vi "Real time state machine - Saccade suppression LED by time.vi"() -> ()   [LabVIEW 2013]
uses:
  <vilib>/Platform/TimedLoop/XDataNode/timing_clust.ctl
  <vilib>/Platform/TimedLoop/XDataNode/nitl_modes.ctl
  <vilib>/Platform/TimedLoop/XDataNode/wakeup.ctl
  <vilib>/DAQmx/write.llb/DAQmx Write (Digital 1D Bool NChan 1Samp 1Line).vi
  <vilib>/DAQmx/read.llb/DAQmx Read (Analog 1D DBL NChan 1Samp).vi
  <vilib>/DAQmx/write.llb/DAQmx Write (Analog DBL 1Chan 1Samp).vi
  <vilib>/platform/TimedLoop/XDataNode/XDataNode.xnode
  <vilib>/Platform/TimedLoop/XDataNode/XDNodeRunTimeDep.lvlib
panel:
  in  "Local port":u16=9091
  in  "Local IP_This computer":string="192.168.137.2"
  out "ABORT":bool
  out "Initial data received":bool
  out "Busy":bool
  out "Trial Done":bool
  in  "Remote port":u16=9090
  in  "Remote IP_Main":string="192.168.137.10"
  out "Trial #":i32=1
  out "Start one trial":bool
  out "RT FIFO (Log)":u32(slide) scale=0.0..50.0
  out "error out":errorcluster
  out "Actual cycle period (uS)":i64=94
  out "# of rewards":i32
  in  "Automatic reward":bool=TRUE
  out "Digital Waveform Graph":digitalwaveform(graph)={"t0"=timestamp(3524542772.3366966 s since 1904-01-01), "dt"=0.0004, "Y"={"transitions"=[], "data"=array25000x3[75000 elements]}, "error"={"status"=FALSE, "code"=37421928, "source"=""}}
  out "shaft encoder":waveform(sgl)(graph)={"t0"=timestamp(3524542772.3366966 s since 1904-01-01), "dt"=0.02, "Y"=array[500 elements]}
  out "Min":dbl
  out "Sec":dbl=47.16078567504883
  out "Trial # (State machine)":u32=1
  out "Current state":T1(ring)=enum."VS"
  out "RT FIFO (DISP)":u32(slide) scale=0.0..50.0
  in  "State machine cycle (uS)":i64=200
  in  "Save file to":string="C:\\ni-rt\\LabVIEW Data\\"
  in  "Display length (S)":sgl=10.0
  in  "RT FIFO size":u32=50
  in  "VS filter period (uS)":i32=500
  out "LED?":bool
  out "Pulse amp 0":sgl
  out "Pulse amp 1":sgl
  out "Pulse delay":sgl
  out "Pulse width":sgl
  out "Pulse period (ms)":sgl
  out "Pulse #":sgl
  out "Reward period (uS)":u32
  out "Reward start delay (uS)":u32
  out "Water duration (uS)":u32=30000
  out "Water refractory period (uS)":u32=500000
  out "Shock duration (uS)":u32=10000
  out "Shock refractory period (uS)":u32=1000000
  out "Trial timeout (uS)":u32=3000000
  out "Lick threshold (V)":fxp<+,32,16>=1.600006103515625
  out "Track eye":bool=TRUE
  out "Allow shock":bool
  out "Allow timeout":bool
  out "Manually give water":bool
  out "Manually give shock":bool
  out "VS threshold (V)":fxp<+,32,16>=0.5
  out "VS type":string="continuous_flash"
  out "File name":string="Test"
  out "Behavior type":string="fullfield"
  out "Save data":bool
  out "Lick reward":bool
  in  "Stop state":bool
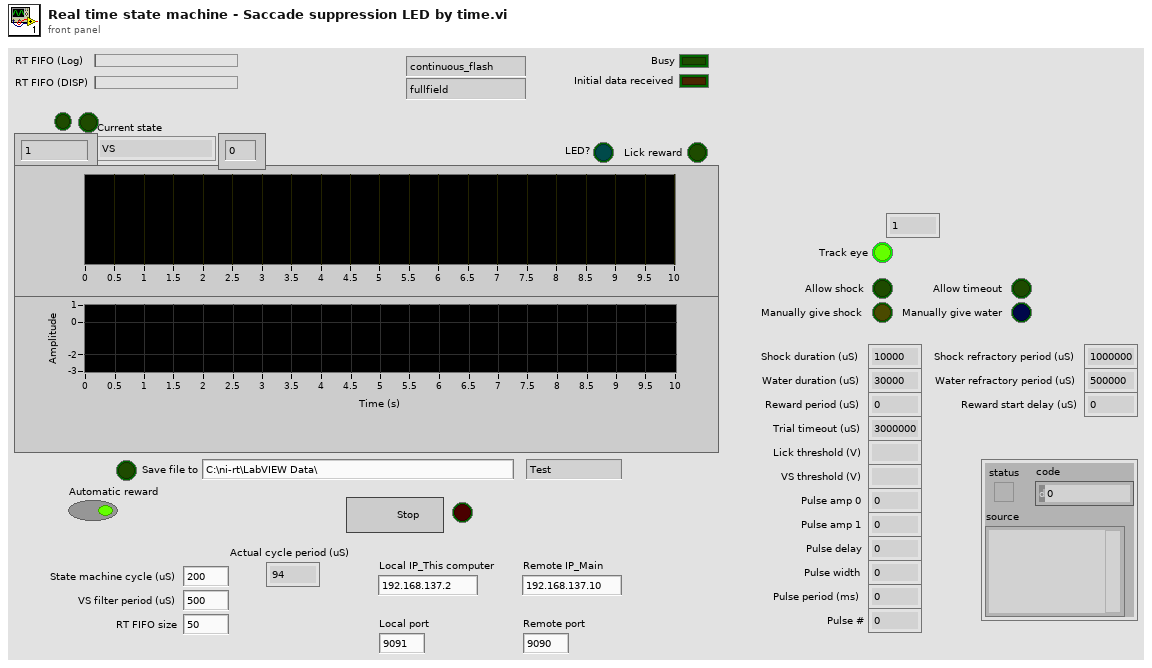
[diagram p1: front panel]
types:
  T1 = enum16{"Idle", "Before VS", "VS", "VS2", "After VS", "Wait for lever press", "Cycle End", "Reward", "Reward Refractory", "Punish", "Punish Refractory", "Exit", "Timeout", "Lick reward"}
  T2 = enum16{"open", "replace", "create", "open or create", "replace or create", "replace or create with confirmation"}
  T3 = typedef "XDNodeRunTimeDep.lvlib/timing_clust.ctl" = cluster{"Expected End [f-1]":u64, "Actual End [f-1]":u64, "Finished Late? [f-1]":bool, "Expected End [i-1]":u64, "Actual End [i-1]":u64, "Finished Late? [i-1]":bool, "Expected Start [i]":u64, "Actual Start [i]":u64, "Expected Start [f]":u64, "Actual Start [f]":u64, "Source Name":string, "Structure Name":string, "Period":i64, "Deadline":i64, "Offset":i64, "Start":i64, "Priority":i32, "Timeout":i32, "Mode":T4, "Wakeup Reason":T5, "Error":errorcluster, "Source Type":string, "Secondary Source Type":string, "Global End Time":u64, "Global Start Time":u64, "Frame Duration":u64, "Iteration Duration":u64, "Assigned CPU":i32, "I/O Scan Engine Mode":u32}
  T4 = typedef "XDNodeRunTimeDep.lvlib/nitl_modes.ctl" = enum32{"No Change", "Process missed periods, maintain original phase", "Discard missed periods, maintain original phase", "Process missed periods, ignore original phase", "Discard missed periods, ignore original phase"}
  T5 = typedef "XDNodeRunTimeDep.lvlib/wakeup.ctl" = enum32{"Normal", "Aborted", "Asynchronous wakeup", "Timing source error", "Timed loop error", "Timeout"}
  T6 = enum16{"big-endian, network order", "native, host order", "little-endian"}
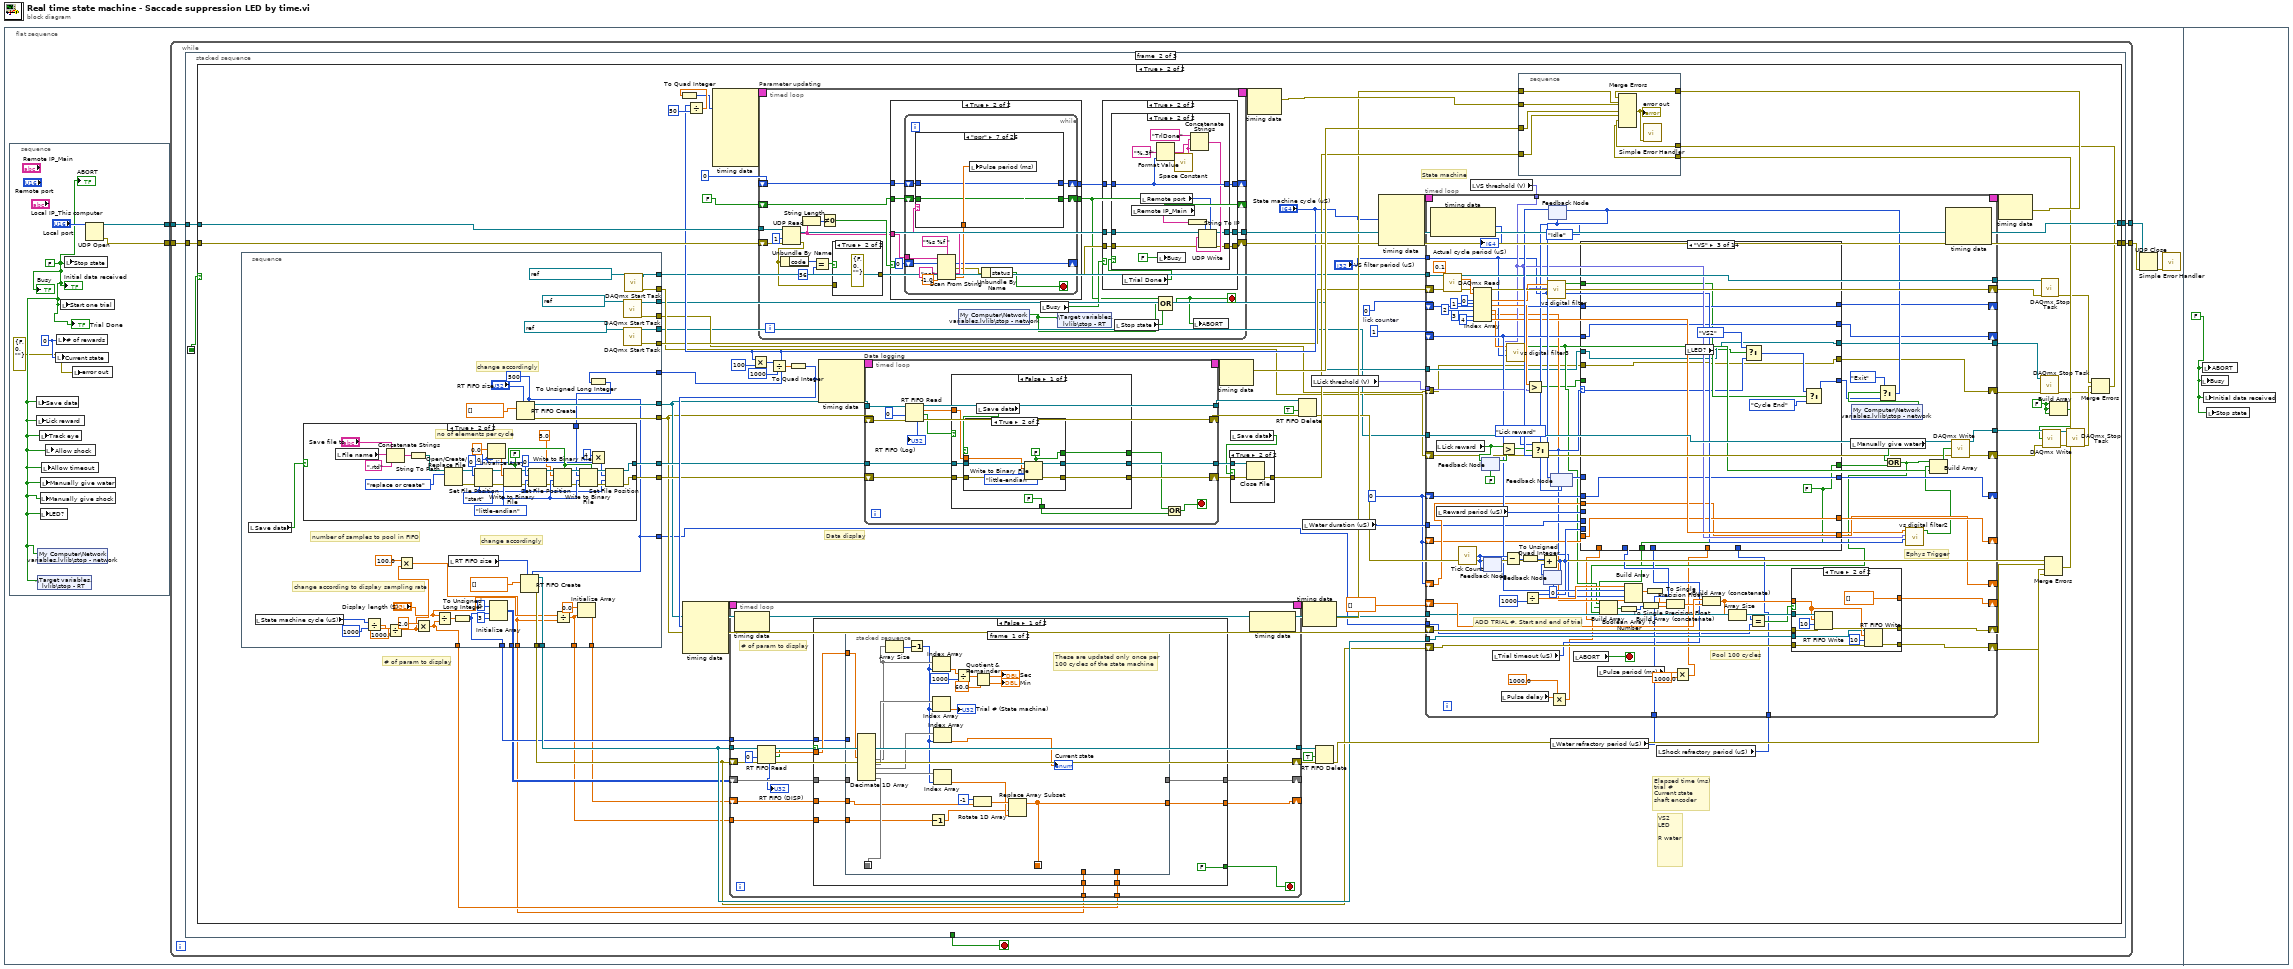
[diagram p0: block diagram]
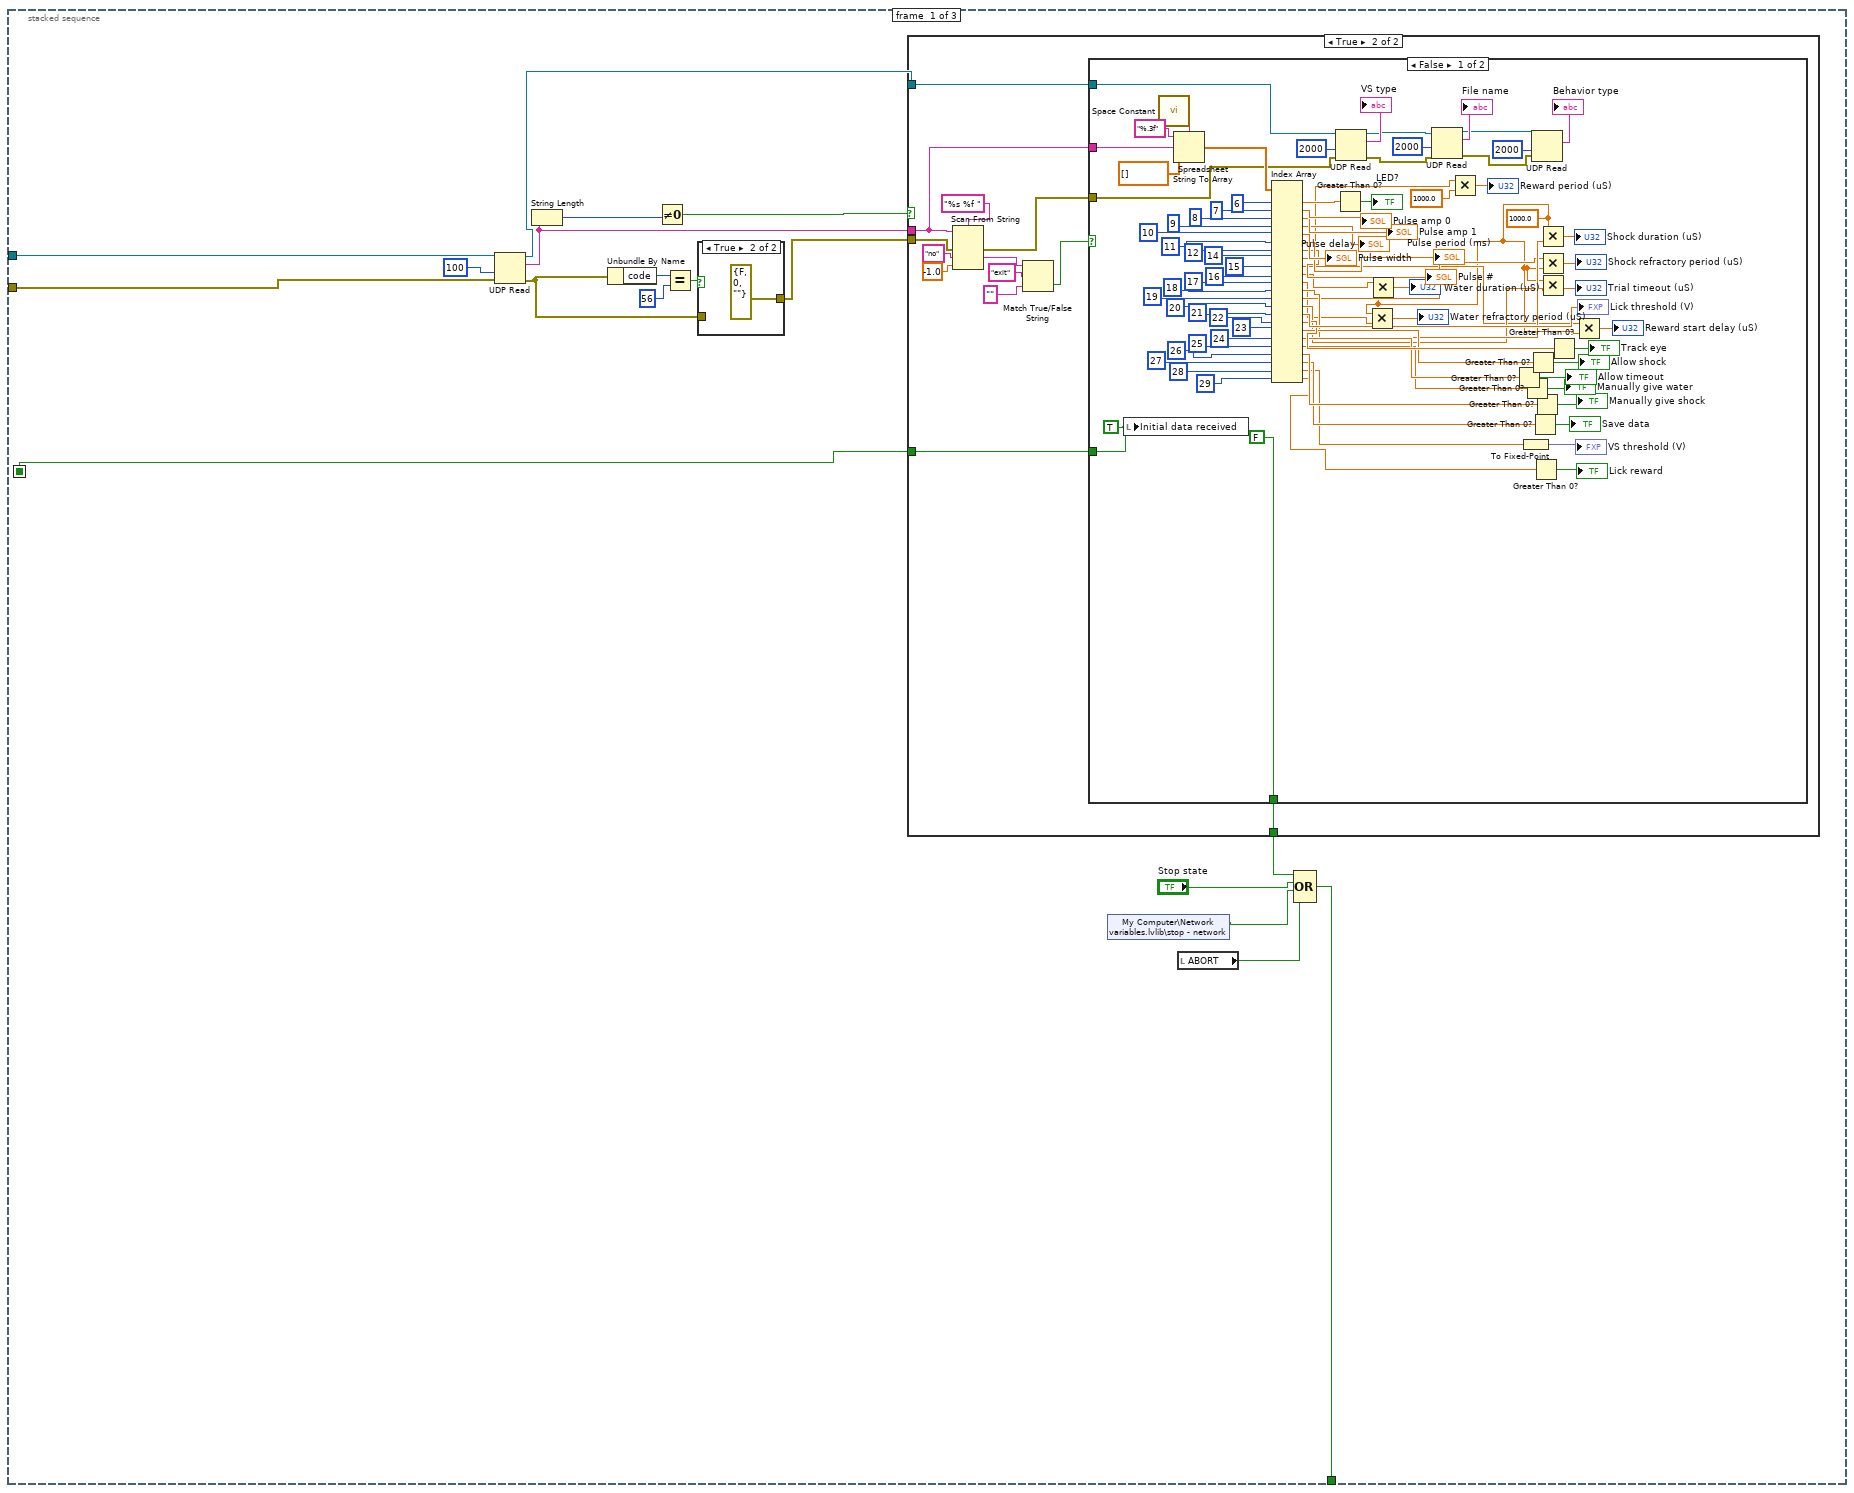
[diagram p2: hidden frame]
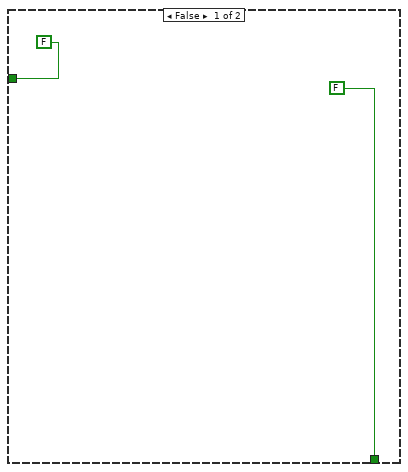
[diagram p3: hidden frame]
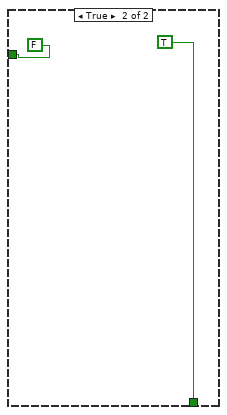
[diagram p4: hidden frame]
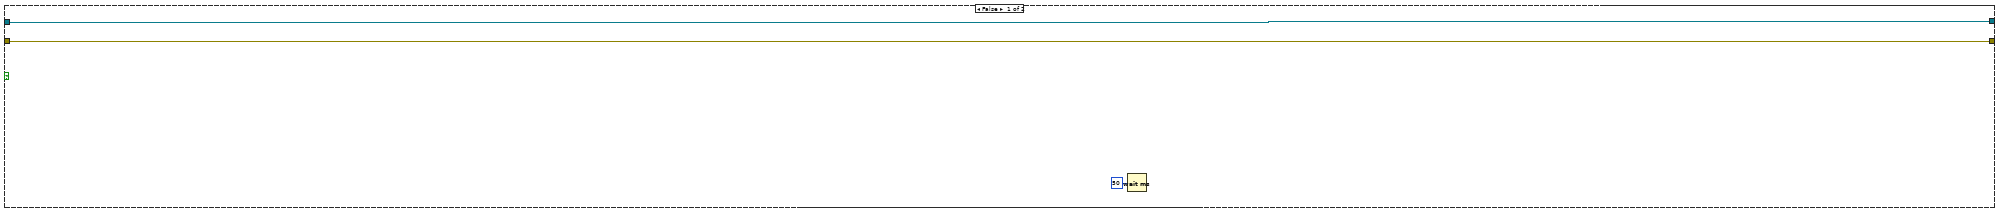
[diagram p6: hidden frame]
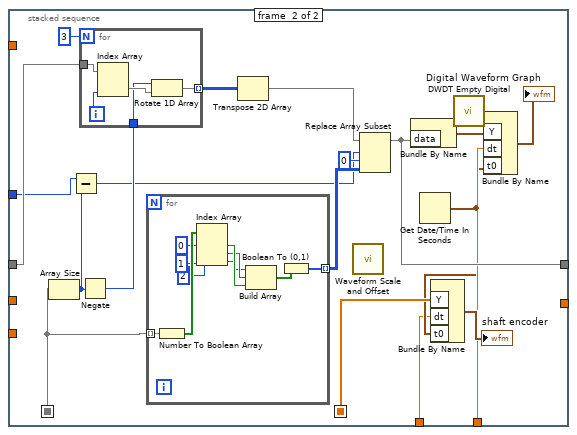
[diagram p9: hidden frame]
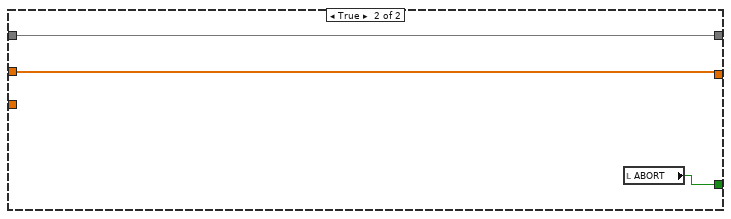
[diagram p10: hidden frame]
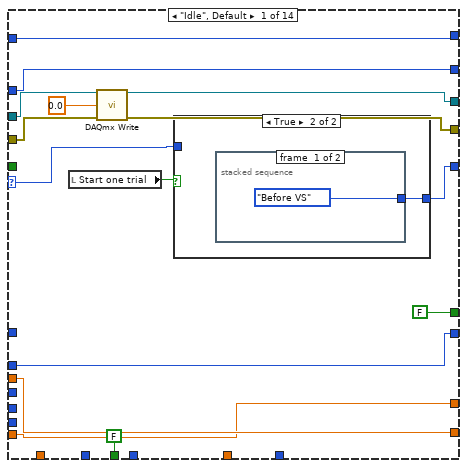
[diagram p11: hidden frame]
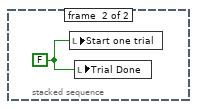
[diagram p13: hidden frame]
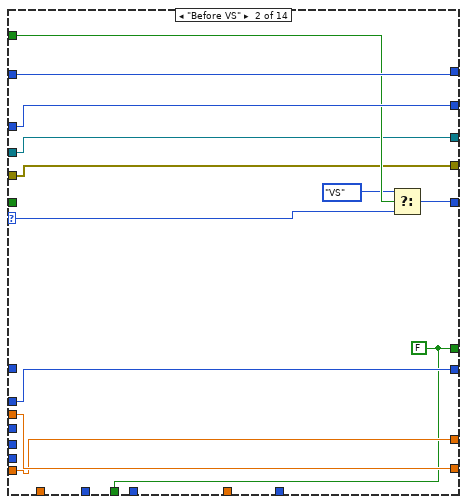
[diagram p14: hidden frame]
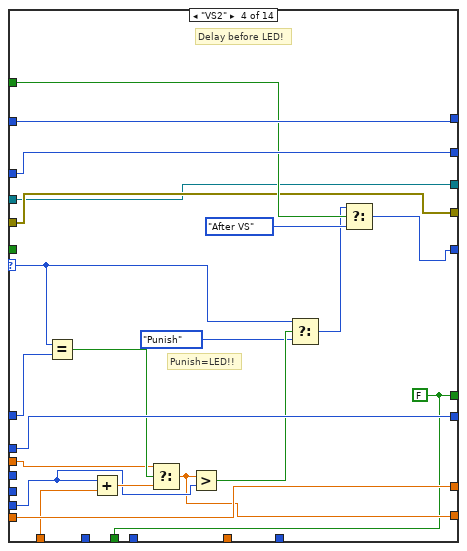
[diagram p15: hidden frame]
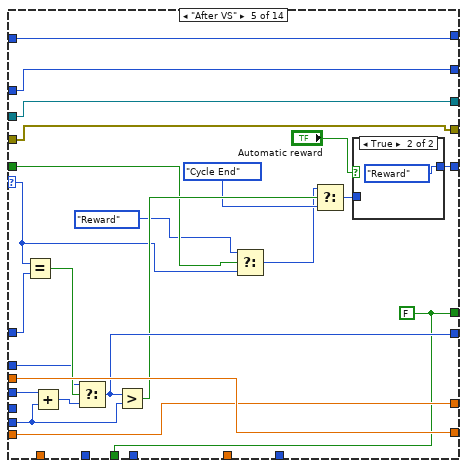
[diagram p16: hidden frame]
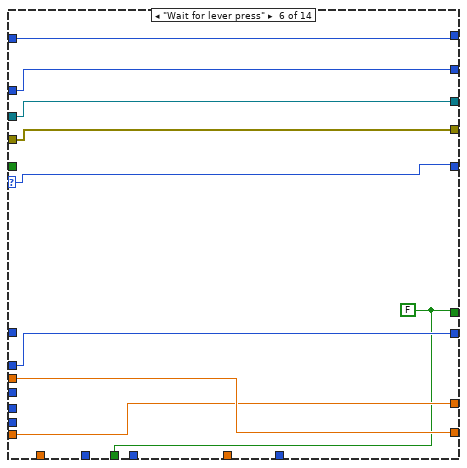
[diagram p18: hidden frame]
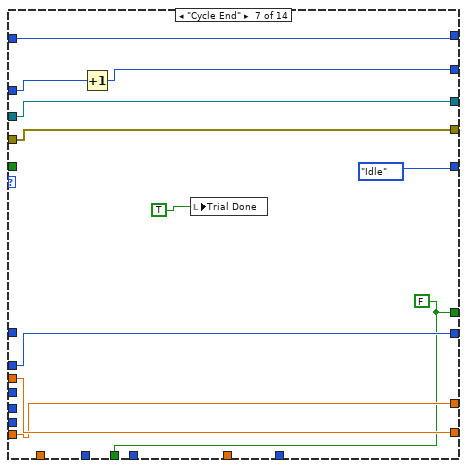
[diagram p19: hidden frame]
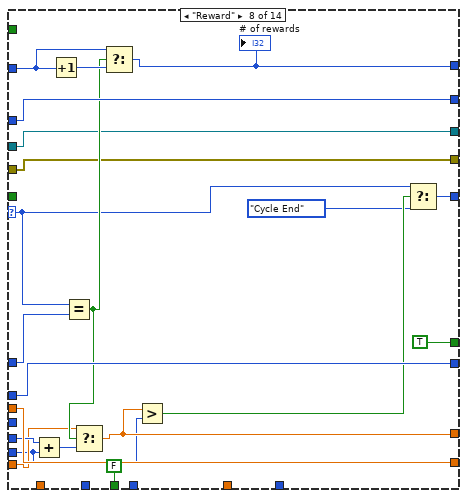
[diagram p20: hidden frame]
diagram:
  n1 = flat-sequence {
    frame #0 {
      n2 = stacked-sequence {
        tunnel: [w998] -> w5
        tunnel: [w997] -> w4
        frame #0 {
          w996 = 0
          w995 = FALSE
          n3 = local write "Save data"(w995) -> ()
          n4 = local write "Lick reward"(w995) -> ()
          n5 = shared-variable "My Computer\\Network variables.lvlib\\stop - network"(w995) -> ()  [unwired: 1 in, 1 out]
          n6 = shared-variable ".\\Target variables.lvlib\\stop - RT"(w995) -> ()  [unwired: 1 in, 1 out]
          n7 = local write "Track eye"(w995) -> ()
          n8 = local write "Manually give shock"(w995) -> ()
          n9 = local write "LED?"(w995) -> ()
          n10 = local write "Manually give water"(w995) -> ()
          n11 = local write "Allow timeout"(w995) -> ()
          n12 = local write "Allow shock"(w995) -> ()
          n13 = local write "Current state"(w996) -> ()
          n14 = local write "# of rewards"(w996) -> ()
          n15 = local write "Start one trial"(w995) -> ()
          n16 = local write "Stop state"(w995) -> ()
          n17 = local write "error out"(errorcluster {"status"=FALSE, "code"=0, "source"=""} ("error out")) -> ()
          n18 = UDP Open(11:"Local port") -> (port=w998:refnum<k16>, 0:w997:errorcluster)  [unwired: 4 in, 1 out]
          "ABORT" <- w995
          "Initial data received" <- w995
          "Busy" <- w995
          "Trial Done" <- w995
        }
      }
      n19 = while {
        tunnel: w5 -> [w10]
        tunnel: w4 -> [w9]
        tunnel: [w8] -> w3
        tunnel: [w7] -> w2
        stop <- w6 stop-if-true
        n20 = stacked-sequence {
          seq-local: [w16 _ _] -> [_ w135 _]
          tunnel: w10 -> [w27 w132 _]
          tunnel: w9 -> [w26 w133 _]
          tunnel: [w15 _ _] -> w6
          tunnel: [_ w134 _] -> w8
          tunnel: [_ w131 _] -> w7
          frame #0 {
            n21 = UDP Read(connection ID=w27, timeout ms (25000)=100, 8:w26) -> (data out=w18:string, error out=w22:errorcluster, 3:w17:refnum<k16>)  [unwired: 1 in, 2 out]
            n22 = String Length(string=w18) -> (length=w21:i32)
            n23 = Unbundle By Name(w22) -> ("code"=w25:i32)
            n24 = Not Equal To 0?(x=w21) -> (x != 0?=w20:bool)
            n25 = Equal?(x=w25, y=56) -> (x = y?=w23:bool)
            n26 = case shown="True" w23 {
              tunnel: w22 -> [w129 _]
              tunnel: [w129 errorcluster {"status"=FALSE, "code"=0, "source"=""} ("error out")] -> w19
              frame False {
              }
              frame True {
              }
            }
            n27 = case shown="True" w20 {
              tunnel: w19 -> [_ w41]
              tunnel: w18 -> [_ w35]
              tunnel: w17 -> [_ w33]
              tunnel: [FALSE w32] -> w14
              tunnel: [FALSE w31] -> w16
              frame False {
              }
              frame True {
                n28 = Scan From String(format string="%s %f ", input string=w35, error in=w41, default 1="no" ("default value 1"), default 2=sgl -1.0 ("default value 1")) -> (error out=w34:errorcluster, output 1=w39:string)  [unwired: 2 in, 2 out]
                n29 = Match True/False String(2:"" ("false string"), 3:"exit" ("true string"), 4:w39) -> (0:w36:bool)  [unwired: 1 out]
                n30 = case shown="False" w36 {
                  tunnel: w35 -> [w123 _]
                  tunnel: w34 -> [w81 _]
                  tunnel: w33 -> [w80 _]
                  tunnel: [FALSE TRUE] -> w32
                  tunnel: [w68 FALSE] -> w31
                  frame False {
                    w49 = sgl 1000.0
                    w68 = TRUE
                    n31 = local write "Initial data received"(w68) -> ()
                    n32 = call <vilib>:"Space Constant.vi"() -> ("String"=w125:string)
                    n33 = Spreadsheet String To Array(delimiter (Tab)=w125, format string="%.3f", spreadsheet string=w123, array type (2D Dbl)=sgl[] []) -> (array=w122:sgl[])
                    n34 = Index Array(array=w122, index #1=6 ("index"), index #2=7 ("index"), index #3=8 ("index"), index #4=9 ("index"), index #5=10 ("index"), index #6=11 ("index"), index #7=12 ("index"), index #8=14 ("index"), index #9=15 ("index"), index #10=16 ("index"), index #11=17 ("index"), index #12=18 ("index"), index #13=19 ("index"), index #14=20 ("index"), index #15=21 ("index"), index #16=22 ("index"), index #17=23 ("index"), index #18=24 ("index"), index #19=25 ("index"), index #20=26 ("index"), index #21=27 ("index"), index #22=28 ("index"), index #23=29 ("index")) -> (element #1=w120:sgl, element #2=→"Pulse amp 0":sgl, element #3=→"Pulse amp 1":sgl, element #4=→"Pulse delay":sgl, element #5=→"Pulse width":sgl, element #6=→"Pulse period (ms)":sgl, element #7=→"Pulse #":sgl, element #8=w64:sgl, element #9=w55:sgl, element #10=w53:sgl, element #11=w51:sgl, element #12=w61:sgl, element #13=w60:sgl, element #14=w57:sgl, element #15=→"Lick threshold (V)":sgl, element #16=w94:sgl, element #17=w91:sgl, element #18=w89:sgl, element #19=w86:sgl, element #20=w84:sgl, element #21=w46:sgl, element #22=w45:sgl, element #23=w44:sgl)
                    n35 = Greater Than 0?(x=w120) -> (x > 0?=→"LED?":bool)
                    n36 = UDP Read(connection ID=w80, timeout ms (25000)=2000, 8:w81) -> (data out=→"VS type":string, error out=w76:errorcluster, 3:w74:refnum<k16>)  [unwired: 1 in, 2 out]
                    n37 = Multiply(x=w49, y=w51) -> (x*y=→"Water refractory period (uS)":sgl)
                    n38 = Multiply(x=w53, y=w49) -> (x*y=→"Water duration (uS)":sgl)
                    n39 = UDP Read(connection ID=w74, timeout ms (25000)=2000, 8:w76) -> (data out=→"File name":string, error out=w72:errorcluster, 3:w71:refnum<k16>)  [unwired: 1 in, 2 out]
                    n40 = Multiply(x=w64, y=sgl 1000.0) -> (x*y=→"Reward period (uS)":sgl)
                    n41 = Greater Than 0?(x=w89) -> (x > 0?=→"Allow timeout":bool)
                    n42 = To Fixed-Point(number=w45) -> (fixed-point=→"VS threshold (V)":fxp<+/-,32,16>)  [unwired: 1 in]
                    n43 = Greater Than 0?(x=w86) -> (x > 0?=→"Manually give water":bool)
                    n44 = Greater Than 0?(x=w91) -> (x > 0?=→"Allow shock":bool)
                    n45 = Greater Than 0?(x=w46) -> (x > 0?=→"Save data":bool)
                    n46 = Greater Than 0?(x=w44) -> (x > 0?=→"Lick reward":bool)
                    n47 = UDP Read(connection ID=w71, timeout ms (25000)=2000, 8:w72) -> (data out=→"Behavior type":string)  [unwired: 1 in, 4 out]
                    n48 = Greater Than 0?(x=w84) -> (x > 0?=→"Manually give shock":bool)
                    n49 = Multiply(x=w49, y=w61) -> (x*y=→"Shock duration (uS)":sgl)
                    n50 = Multiply(x=w60, y=w49) -> (x*y=→"Shock refractory period (uS)":sgl)
                    n51 = Multiply(x=w49, y=w57) -> (x*y=→"Trial timeout (uS)":sgl)
                    n52 = Greater Than 0?(x=w94) -> (x > 0?=→"Track eye":bool)
                    n53 = Multiply(x=w55, y=w49) -> (x*y=→"Reward start delay (uS)":sgl)
                  }
                  frame True {
                  }
                }
              }
            }
            n54 = shared-variable "My Computer\\Network variables.lvlib\\stop - network"() -> (w11:bool)  [unwired: 1 in, 1 out]
            n55 = local read "ABORT"() -> (w12:bool)
            n56 = Compound Arithmetic op=OR(w14, "Stop state", w11, w12) -> (w15:bool)
          }
          frame #1 {
            n57 = case shown="True" w135 {
              tunnel: w133 -> [w138 w215]
              tunnel: [w138 w207] -> w134
              tunnel: w132 -> [w137 w214]
              tunnel: [w137 w206] -> w131
              frame False {
                n58 = Wait (ms)(milliseconds to wait=u32 50) -> ()  [unwired: 1 out]
              }
              frame True {
                w159 = FALSE
                w195 = 0  # lick counter
                w152 = 0
                # "VS2\nLED\n\nR water"
                # "# of param to display"
                # "Data display"
                # "Elapsed time (ms)\ntrial #\nCurrent state\nshaft encoder"
                # "State machine"
                n59 = stacked-sequence {
                  tunnel: [w267] -> w180
                  tunnel: [w266] -> w179
                  tunnel: [w263] -> w178
                  tunnel: [w262] -> w177
                  tunnel: [w248] -> w160
                  tunnel: [w243] -> w176
                  tunnel: [w254] -> w175
                  tunnel: "State machine cycle (uS)" -> [w247]
                  tunnel: [w251] -> w173
                  tunnel: [w250] -> w172
                  tunnel: [w245] -> w151
                  tunnel: [w242] -> w150
                  tunnel: [w238] -> w149
                  tunnel: [w237] -> w148
                  tunnel: [w235] -> w144
                  tunnel: [w234] -> w143
                  tunnel: [w232] -> w142
                  tunnel: [w231] -> w141
                  tunnel: [w229] -> w140
                  tunnel: [w228] -> w139
                  frame #0 {
                    w245 = u32 500 ("elements in array (1)")
                    # "number of samples to pool in FIFO"
                    # "change according to display sampling rate"
                    # "change accordingly"
                    # "change accordingly"
                    n60 = local read "Save data"() -> (w268:bool)
                    n61 = local read "State machine cycle (uS)"() -> (w255:i64)
                    n62 = Divide(x=w255, y=u32 1000) -> (x/y=w257:dbl)
                    n63 = Divide(x=w257, y=1000.0) -> (x/y=w240:dbl)
                    n64 = Multiply(x=100.0, y=w240) -> (x*y=w238:dbl)
                    n65 = Multiply(x=2.0, y=w240) -> (x*y=w248:dbl)
                    n66 = Divide(x="Display length (S)", y=w248) -> (x/y=w260:dbl)
                    n67 = local read "RT FIFO size"() -> (w265:u32)
                    n68 = To Unsigned Long Integer(number=w260) -> (unsigned 32bit integer=w243:u32)
                    n69 = Initialize Array(u8 0 ("element"), w243, 3 ("dimension size")) -> (w254:u8[][])
                    n70 = RT FIFO Create(1:sgl[] [], 4:"RT FIFO size", 6:w245) -> (8:w251:refnum<k33>, 11:w250:errorcluster)  [unwired: 5 in, 1 out]
                    n71 = RT FIFO Create(1:sgl[] [], 4:w265, 6:w245) -> (8:w263:refnum<k33>, 11:w262:errorcluster)  [unwired: 5 in, 1 out]
                    n72 = Divide(x="Display length (S)", y=w238) -> (x/y=w237:dbl)
                    n73 = Initialize Array(sgl 0.0 ("element"), w237) -> (w242:sgl[])
                    n74 = To Unsigned Long Integer(number=w247) -> (unsigned 32bit integer=w246:u32)
                    n75 = case shown="True" w268 {
                      tunnel: [_ w272] -> w267
                      tunnel: [_ w271] -> w266
                      tunnel: w246 -> [_ w270]
                      frame False {
                      }
                      frame True {
                        w293 = FALSE
                        w286 = 10 ("dimension size")
                        w294 = T6."little-endian" ("byte order (0:big-endian, network order)")
                        w285 = enum16{"start", "end", "current"}."start" ("from (0:start)")
                        # "no of elements per cycle"
                        n76 = local read "File name"() -> (w296:string)
                        n77 = Concatenate Strings("Save file to", w296, ".rtd" ("string")) -> (w299:string)
                        n78 = String To Path(string=w299) -> (path=w300:path)
                        n79 = Open/Create/Replace File(file path (use dialog)=w300, operation (0:open)=T2."replace or create") -> (refnum out=w273:refnum<file>, error out=w274:errorcluster)  [unwired: 4 in, 1 out]
                        n80 = Set File Position(offset (in bytes) (0)=i64 0, refnum=w273, from (0:start)=w285, error in=w274) -> (refnum out=w276:refnum<file>, error out=w277:errorcluster)
                        n81 = Initialize Array(sgl 0.0 ("element"), w286) -> (w279:sgl[])
                        n82 = Write to Binary File(file (use dialog)=w276, data=w279, error in=w277, 5:w293, 9:w294) -> (refnum out=w281:refnum<file>, error out=w280:errorcluster)  [unwired: 1 in, 1 out]
                        n83 = Set File Position(offset (in bytes) (0)=i64 0, refnum=w281, from (0:start)=w285, error in=w280) -> (refnum out=w283:refnum<file>, error out=w284:errorcluster)
                        n84 = Write to Binary File(file (use dialog)=w283, data=sgl 5.0, error in=w284, 5:w293, 9:w294) -> (refnum out=w291:refnum<file>, error out=w289:errorcluster)  [unwired: 1 in, 1 out]
                        n85 = Write to Binary File(file (use dialog)=w291, data=w270, error in=w289, 5:w293, 9:w294) -> (refnum out=w292:refnum<file>, error out=w290:errorcluster)  [unwired: 1 in, 1 out]
                        n86 = Multiply(x=4, y=w286) -> (x*y=w288:i32)
                        n87 = Set File Position(offset (in bytes) (0)=w288, refnum=w292, from (0:start)=w285, error in=w290) -> (refnum out=w271:refnum<file>, error out=w272:errorcluster)
                      }
                    }
                    n88 = call <vilib>:"DAQmx Start Task.vi"("task/channels in"=refnum<k21> "LED analog out" ("DAQmx Task Name")) -> ("task out"=w232:refnum<k21>, "error out"=w231:errorcluster)  [unwired: 13 in]
                    n89 = call <vilib>:"DAQmx Start Task.vi"("task/channels in"=refnum<k21> "Digital_write_saccade" ("DAQmx Task Name")) -> ("task out"=w229:refnum<k21>, "error out"=w228:errorcluster)  [unwired: 13 in]
                    n90 = call <vilib>:"DAQmx Start Task.vi"("task/channels in"=refnum<k21> "Analog_read_saccade" ("DAQmx Task Name")) -> ("task out"=w235:refnum<k21>, "error out"=w234:errorcluster)  [unwired: 13 in]
                  }
                }
                n91 = Divide(x="State machine cycle (uS)", y=i64 50) -> (x/y=w185:dbl)
                n92 = To Quad Integer(1:w185) -> (0:w184:i64)
                n93 = node-c288 ("Input Node")(w184) -> (w223:T3)  [unwired: 6 in]
                n94 = Multiply(x="State machine cycle (uS)", y=u32 100) -> (x*y=w188:i64)
                n95 = timed-loop "Parameter updating" {
                  timing: w223 -> [_]
                  timing-out: [_] -> w222
                  tunnel: w214 -> [w831]
                  shift-right: [w816] -> w207
                  shift-left: w215 -> [w832]
                  shift-right: [w819] -> _
                  shift-left: 0 -> [w822]
                  tunnel: [w815] -> w206
                  shift-right: [w813] -> _
                  shift-left: FALSE -> [w823]
                  stop <- w814 stop-if-true
                  n96 = UDP Read(connection ID=w831, timeout ms (25000)=1, 8:w832) -> (data out=w824:string, error out=w827:errorcluster, 3:w817:refnum<k16>)  [unwired: 1 in, 2 out]
                  n97 = Unbundle By Name(w827) -> ("code"=w830:i32)
                  n98 = String Length(string=w824) -> (length=w826:i32)
                  n99 = Equal?(x=w830, y=56) -> (x = y?=w828:bool)
                  n100 = Not Equal To 0?(x=w826) -> (x != 0?=w825:bool)
                  n101 = case shown="True" w828 {
                    tunnel: w827 -> [w984 _]
                    tunnel: [w984 errorcluster {"status"=FALSE, "code"=0, "source"=""} ("error out")] -> w818
                    frame False {
                    }
                    frame True {
                    }
                  }
                  n102 = case shown="True" w825 {
                    tunnel: w824 -> [_ w867]
                    tunnel: w823 -> [w860 w866]
                    tunnel: w822 -> [w861 w865]
                    tunnel: [w861 w864] -> w820
                    tunnel: [w860 w863] -> w813
                    frame False {
                    }
                    frame True {
                      n103 = while {
                        tunnel: w867 -> [w879]
                        shift-right: [w875] -> w863
                        shift-left: w866 -> [w876]
                        shift-right: [w874] -> w864
                        shift-left: w865 -> [w873]
                        shift-right: [w869] -> _
                        shift-left: u32 0 -> [w870]
                        stop <- w871 stop-if-true
                        n104 = Scan From String(format string="%s %f ", input string=w879, initial scan location=w870, default 1="no" ("default value 1"), default 2=-1.0 ("default value 2")) -> (offset past scan=w869:u32, error out=w872:errorcluster, output 1=w878:string, output 2=w877:dbl)  [unwired: 1 in, 1 out]
                        n105 = case shown="\"ppr\"" w878 {
                          tunnel: w877 -> [_ w886 w890 w893 w896 w899 w902 w905 w907 w911 w916 w922 w927 w932 w937 w943 w946 w950 w955 w958 w962 w966 w969 w973 _ _]
                          tunnel: w876 -> [w883 w884 w888 w891 w894 w897 w900 w903 w909 w914 w919 w924 w929 w934 w939 w941 w944 w948 w952 w956 w960 w964 w970 w974 w977 w982]
                          tunnel: [w883 w884 w888 w891 w894 w897 w900 w903 w909 w914 w919 w924 w929 w934 w939 w941 w944 w948 w952 w956 w960 w964 w970 w974 w977 w981] -> w875
                          tunnel: [w882 w885 w889 w892 w895 w898 w901 w904 w910 w915 w920 w925 w930 w935 w940 w942 w945 w949 w953 w957 w961 w965 w971 w975 w978 w980] -> w874
                          tunnel: w873 -> [w882 w885 w889 w892 w895 w898 w901 w904 w910 w915 w920 w925 w930 w935 w940 w942 w945 w949 w953 w957 w961 w965 w971 w975 w979 w980]
                          frame "no", Default {
                          }
                          frame "led" {
                            n106 = Greater Than 0?(x=w886) -> (x > 0?=w887:bool)
                            n107 = local write "LED?"(w887) -> ()
                          }
                          frame "pai" {
                            n108 = local write "Pulse amp 0"(w890) -> ()
                          }
                          frame "paf" {
                            n109 = local write "Pulse amp 1"(w893) -> ()
                          }
                          frame "pdl" {
                            n110 = local write "Pulse delay"(w896) -> ()
                          }
                          frame "pwd" {
                            n111 = local write "Pulse width"(w899) -> ()
                          }
                          frame "ppr" {
                            n112 = local write "Pulse period (ms)"(w902) -> ()
                          }
                          frame "pnm" {
                            n113 = local write "Pulse #"(w905) -> ()
                          }
                          frame "rwp" {
                            n114 = Multiply(x=1000.0, y=w907) -> (x*y=w906:dbl)
                            n115 = local write "Reward period (uS)"(w906) -> ()
                          }
                          frame "rwd" {
                            n116 = Multiply(x=1000.0, y=w911) -> (x*y=w912:dbl)
                            n117 = local write "Reward start delay (uS)"(w912) -> ()
                          }
                          frame "wdr" {
                            n118 = Multiply(x=1000.0, y=w916) -> (x*y=w917:dbl)
                            n119 = local write "Water duration (uS)"(w917) -> ()
                          }
                          frame "wre" {
                            n120 = Multiply(x=1000.0, y=w922) -> (x*y=w921:dbl)
                            n121 = local write "Water refractory period (uS)"(w921) -> ()
                          }
                          frame "shd" {
                            n122 = Multiply(x=1000.0, y=w927) -> (x*y=w926:dbl)
                            n123 = local write "Shock duration (uS)"(w926) -> ()
                          }
                          frame "shr" {
                            n124 = Multiply(x=1000.0, y=w932) -> (x*y=w931:dbl)
                            n125 = local write "Shock refractory period (uS)"(w931) -> ()
                          }
                          frame "tto" {
                            n126 = Multiply(x=1000.0, y=w937) -> (x*y=w936:dbl)
                            n127 = local write "Trial timeout (uS)"(w936) -> ()
                          }
                          frame "lkt" {
                            n128 = local write "Lick threshold (V)"(w943) -> ()
                          }
                          frame "etk" {
                            n129 = Greater Than 0?(x=w946) -> (x > 0?=w947:bool)
                            n130 = local write "Track eye"(w947) -> ()
                          }
                          frame "ash" {
                            n131 = Greater Than 0?(x=w950) -> (x > 0?=w951:bool)
                            n132 = local write "Allow shock"(w951) -> ()
                          }
                          frame "ato" {
                            n133 = Greater Than 0?(x=w955) -> (x > 0?=w954:bool)
                            n134 = local write "Allow timeout"(w954) -> ()
                          }
                          frame "gwt" {
                            n135 = Greater Than 0?(x=w958) -> (x > 0?=w959:bool)
                            n136 = local write "Manually give water"(w959) -> ()
                          }
                          frame "gsh" {
                            n137 = Greater Than 0?(x=w962) -> (x > 0?=w963:bool)
                            n138 = local write "Manually give shock"(w963) -> ()
                          }
                          frame "sav" {
                            n139 = Greater Than 0?(x=w966) -> (x > 0?=w967:bool)
                            n140 = local write "Save data"(w967) -> ()
                          }
                          frame "vsh" {
                            n141 = To Fixed-Point(number=w969) -> (fixed-point=w968:fxp<+/-,32,16>)  [unwired: 1 in]
                            n142 = local write "VS threshold (V)"(w968) -> ()
                          }
                          frame "rew" {
                            n143 = Greater Than 0?(x=w973) -> (x > 0?=w972:bool)
                            n144 = local write "Lick reward"(w972) -> ()
                          }
                          frame "start" {
                            w976 = TRUE
                            n145 = Increment(x=w979) -> (x+1=w978:i32)
                            "Trial #" <- w978
                            n146 = local write "Busy"(w976) -> ()
                            "Start one trial" <- w976
                          }
                          frame "stop" {
                            n147 = Or(x=w982, y=TRUE) -> (x .or. y?=w981:bool)
                          }
                        }
                        n148 = Unbundle By Name(w872) -> ("status"=w871:bool)
                      }
                    }
                  }
                  n149 = shared-variable "My Computer\\Network variables.lvlib\\stop - network"() -> (w811:bool)  [unwired: 1 in, 1 out]
                  n150 = local read "Busy"() -> (w821:bool)
                  n151 = shared-variable ".\\Target variables.lvlib\\stop - RT"(w811) -> ()  [unwired: 1 in, 1 out]
                  n152 = case shown="True" w821 {
                    tunnel: w820 -> [w835 w841]
                    tunnel: [w835 w840] -> w819
                    tunnel: w818 -> [w833 w839]
                    tunnel: w817 -> [w834 w838]
                    tunnel: [w833 w837] -> w816
                    tunnel: [w834 w836] -> w815
                    frame False {
                    }
                    frame True {
                      n153 = local read "Trial Done"() -> (w842:bool)
                      n154 = case shown="True" w842 {
                        tunnel: [w845 w853] -> w840
                        tunnel: w841 -> [w845 w853]
                        tunnel: w839 -> [w844 w850]
                        tunnel: w838 -> [w843 w849]
                        tunnel: [w844 w847] -> w837
                        tunnel: [w843 w846] -> w836
                        frame False {
                        }
                        frame True {
                          n155 = local read "Remote IP_Main"() -> (w858:string)
                          n156 = local read "Remote port"() -> (w857:u16)
                          n157 = Format Value(format string="%.3f", value (0)=w853) -> (output string=w852:string)  [unwired: 1 in]
                          n158 = local write "Busy"(FALSE) -> ()
                          n159 = call <vilib>:"Space Constant.vi"() -> ("String"=w855:string)
                          n160 = String To IP(1:w858) -> (0:w859:u32)
                          n161 = Concatenate Strings("TrlDone" ("data in"), w855, w852, w855) -> (w851:string)
                          n162 = UDP Write(address=w859, port or service name=w857, connection ID=w849, data in=w851, 8:w850) -> (error out=w847:errorcluster, 3:w846:refnum<k16>)  [unwired: 1 in]
                        }
                      }
                    }
                  }
                  n163 = local read "Stop state"() -> (w812:bool)
                  n164 = Compound Arithmetic op=OR(w813, w811, w812) -> (w814:bool)
                  n165 = local write "ABORT"(w814) -> ()
                }
                n166 = Divide(x=w188, y=u32 1000) -> (x/y=w183:dbl)
                n167 = To Quad Integer(1:w183) -> (0:w182:i64)
                n168 = node-c288(w182) -> (w209:T3)  [unwired: 3 in]
                n169 = timed-loop {
                  timing: w209 -> [_]
                  timing-out: [_] -> w208
                  shift-right: [w314] -> w193
                  shift-left: w177 -> [w315]
                  tunnel: w178 -> [w317]
                  tunnel: [w316] -> w194
                  tunnel: w176 -> [w309]
                  shift-right: [w308] -> _
                  shift-left: w175 -> [w310]
                  tunnel: w160 -> [w307]
                  shift-right: [w303] -> _
                  shift-left: w150 -> [w304]
                  tunnel: w149 -> [w302]
                  tunnel: w148 -> [w301]
                  stop <- w305 stop-if-true
                  # "# of param to display"
                  n170 = node-c288() -> ()  [unwired: 1 in, 1 out]
                  n171 = RT FIFO Read(0:w317, 2:0 ("timeout in ms (0)"), 3:w315) -> (7:→"RT FIFO (DISP)":u32, 8:w316:refnum<k33>, 9:w312:sgl[], 10:w311:bool, 11:w314:errorcluster)  [unwired: 1 in]
                  n172 = case shown="False" w311 {
                    tunnel: w312 -> [w327 _]
                    tunnel: w310 -> [w326 w388]
                    tunnel: w309 -> [w325 _]
                    tunnel: [w324 w388] -> w308
                    tunnel: w307 -> [w323 _]
                    tunnel: [FALSE w387] -> w305
                    tunnel: w304 -> [w321 w386]
                    tunnel: [w320 w386] -> w303
                    tunnel: w302 -> [w319 _]
                    tunnel: w301 -> [w318 _]
                    frame False {
                      n173 = stacked-sequence {
                        seq-local: [w337 _] -> [_ w367]
                        seq-local: [w329 _] -> [_ w353]
                        tunnel: w327 -> [w350 _]
                        tunnel: w326 -> [_ w369]
                        tunnel: w325 -> [_ w362]
                        tunnel: [_ w359] -> w324
                        tunnel: w323 -> [_ w354]
                        tunnel: w321 -> [w334 _]
                        tunnel: [w329 _] -> w320
                        tunnel: w319 -> [_ w351]
                        tunnel: w318 -> [w328 _]
                        frame #0 {
                          # "These are updated only once per \n100 cycles of the state machine"
                          n174 = Decimate 1D Array(w350) -> (w339:sgl[], w340:sgl[], w341:sgl[], w336:sgl[], w337:sgl[])  [unwired: 5 out]
                          n175 = Array Size(array=w339) -> (size(s)=w349:i32)
                          n176 = Decrement(x=w349) -> (x-1=w335:i32)
                          n177 = Decrement(x=w328) -> (x-1=w330:dbl)
                          n178 = Index Array(array=w339, index=w335) -> (element=w348:sgl)
                          n179 = Index Array(array=w340, index=w335) -> (element=→"Trial # (State machine)":sgl)
                          n180 = Index Array(array=w341, index=w335) -> (element=→"Current state":sgl)
                          n181 = Index Array(array=w336, index=w335) -> (element=w332:sgl)
                          n182 = Divide(x=w348, y=u32 1000) -> (x/y=w346:sgl)
                          n183 = Rotate 1D Array(1:w334, 2:-1 ("n")) -> (0:w333:sgl[])
                          n184 = Quotient & Remainder(x=w346, y=60.0) -> (x-y*floor(x/y)=→"Sec":dbl, floor(x/y)=→"Min":dbl)
                          n185 = Replace Array Subset(array=w333, new element=w332, index=w330) -> (w329:sgl[])
                        }
                        frame #1 {
                          n186 = Array Size(array=w367) -> (size(s)=w361:i32)
                          n187 = Subtract(x=w362, y=w361) -> (x-y=w360:u32)
                          n188 = Negate(x=w361) -> (-x=w368:i32)
                          n189 = for {
                            N: 3 -> [_]
                            tunnel: w369 -> [w385]
                            tunnel: w368 -> [w382]
                            tunnel: [w381] -> w365 mode=indexing
                            i -> [w384]
                            n190 = Index Array(array=w385, index (col)=w384) -> (element=w383:u8[])  [unwired: 1 in]
                            n191 = Rotate 1D Array(1:w383, 2:w382) -> (0:w381:u8[])
                          }
                          n192 = for {
                            tunnel: w367 -> [w380] mode=indexing
                            tunnel: [w374] -> w366 mode=indexing
                            n193 = Number To Boolean Array(number=w380) -> (Boolean array=w379:bool[])
                            n194 = Index Array(array=w379, index #1=0 ("index"), index #2=1 ("index"), index #3=2 ("index")) -> (element #1=w373:bool, element #2=w372:bool, element #3=w371:bool)
                            n195 = Build Array(w371, w372, w373) -> (w375:bool[])
                            n196 = Boolean To (0,1)(Boolean=w375) -> (0, 1=w374:i16[])
                          }
                          n197 = Transpose 2D Array(2D array=w365) -> (transposed array=w364:u8[][])
                          n198 = call <vilib>:"Waveform Scale and Offset.vi"() -> ()  [unwired: 10 in, 2 out]
                          n199 = Replace Array Subset(array=w364, new element=w366, index (row)=w360, index (col)=0 ("disabled index (col)")) -> (w359:u8[][])
                          n200 = Bundle By Name("data"=w359) -> (w358:digitaldata)  [unwired: 1 in]
                          n201 = Get Date/Time In Seconds() -> (seconds since 1Jan1904=w352:timestamp)
                          n202 = Bundle By Name("Y"=w353, "dt"=w351, "t0"=w352) -> (→"shaft encoder":waveform(sgl))  [unwired: 1 in]
                          n203 = call <vilib>:"DWDT Empty Digital.vi"() -> ("digital waveform out"=w357:digitalwaveform)  [unwired: 5 in]
                          n204 = Bundle By Name(cluster=w357, "Y"=w358, "dt"=w354, "t0"=w352) -> (→"Digital Waveform Graph":digitalwaveform)
                        }
                      }
                    }
                    frame True {
                      n205 = local read "ABORT"() -> (w387:bool)
                    }
                  }
                  n206 = node-c288() -> ()  [unwired: 1 in, 1 out]
                }
                n207 = node-c288 ("Input Node")(w182) -> (w221:T3)  [unwired: 2 in]
                n208 = timed-loop "Data logging" {
                  timing: w221 -> [_]
                  timing-out: [_] -> w220
                  tunnel: [w780] -> w216
                  tunnel: w179 -> [w778]
                  tunnel: w173 -> [w775]
                  shift-right: [w774] -> w198
                  shift-left: w172 -> [w776]
                  tunnel: [w772] -> w196
                  shift-right: [w779] -> w217
                  shift-left: w180 -> [w777]
                  stop <- w768 stop-if-true
                  n209 = RT FIFO Read(0:w775, 2:0 ("timeout in ms (0)"), 3:w776) -> (7:→"RT FIFO (Log)":u32, 8:w772:refnum<k33>, 9:w770:sgl[], 10:w771:bool, 11:w774:errorcluster)  [unwired: 1 in]
                  n210 = case shown="False" w771 {
                    tunnel: [w788 w801] -> w780
                    tunnel: [w787 w802] -> w779
                    tunnel: w778 -> [w786 w801]
                    tunnel: w777 -> [w785 w802]
                    tunnel: w770 -> [w783 _]
                    tunnel: [FALSE w799] -> w766
                    tunnel: [w781 FALSE] -> w767
                    frame False {
                      n211 = local read "Save data"() -> (w784:bool)
                      n212 = case shown="True" w784 {
                        tunnel: [w791 w798] -> w788
                        tunnel: [w790 w797] -> w787
                        tunnel: w786 -> [w791 w796]
                        tunnel: w785 -> [w790 w795]
                        tunnel: w783 -> [_ w794]
                        tunnel: [w789 w792] -> w781
                        frame False {
                          n213 = local read "ABORT"() -> (w789:bool)
                        }
                        frame True {
                          w792 = FALSE
                          n214 = Write to Binary File(file (use dialog)=w796, data=w794, error in=w795, 5:w792, 9:T6."little-endian" ("byte order (0:big-endian, network order)")) -> (refnum out=w798:refnum<file>, error out=w797:errorcluster)  [unwired: 1 in, 1 out]
                        }
                      }
                    }
                    frame True {
                      n215 = local read "ABORT"() -> (w799:bool)
                    }
                  }
                  n216 = Or(x=w767, y=w766) -> (x .or. y?=w768:bool)
                }
                n217 = node-c288 ("Output Node")(w220) -> (w219:errorcluster)
                n218 = local read "Save data"() -> (w169:bool)
                n219 = case shown="True" w169 {
                  tunnel: w217 -> [w224 w227]
                  tunnel: w216 -> [_ w226]
                  tunnel: [w224 w225] -> w205
                  frame False {
                  }
                  frame True {
                    n220 = Close File(refnum=w226, error in=w227) -> (error out=w225:errorcluster)  [unwired: 1 out]
                  }
                }
                n221 = node-c288 ("Output Node")(w222) -> (w218:errorcluster)
                n222 = RT FIFO Delete(0:w196, 2:TRUE ("force destroy? (F)"), 3:w198) -> (11:w197:errorcluster)
                n223 = node-c288(w208) -> (w204:errorcluster)
                n224 = local read "Water duration (uS)"() -> (w155:u32)
                n225 = local read "Lick threshold (V)"() -> (w156:fxp<+,32,16>)
                n226 = RT FIFO Delete(0:w194, 2:TRUE ("force destroy? (F)"), 3:w193) -> (11:w192:errorcluster)
                n227 = node-c288("State machine cycle (uS)") -> (w211:T3)  [unwired: 3 in]
                n228 = local read "VS threshold (V)"() -> (w157:fxp<+,32,16>)
                n229 = local read "Water refractory period (uS)"() -> (w153:u32)
                n230 = local read "Shock refractory period (uS)"() -> (w154:u32)
                n231 = timed-loop {
                  timing: w211 -> [_]
                  timing-out: [_] -> w210
                  shift-right: [w434] -> _
                  shift-left: w152 -> [w446]
                  shift-right: [w436] -> _
                  shift-left: 1 -> [w447]
                  shift-right: [w433] -> _
                  shift-left: w152 -> [w441]
                  tunnel: w173 -> [w478]
                  shift-right: [w477] -> w200
                  shift-left: w172 -> [w476]
                  shift-right: [w437] -> _
                  shift-left: w195 -> [w448]
                  tunnel: w178 -> [w473]
                  shift-right: [w471] -> w191
                  shift-left: w177 -> [w472]
                  shift-right: [w474] -> _
                  shift-left: sgl[] [] ("array type (2D Dbl)") -> [w479]
                  tunnel: w144 -> [w464]
                  tunnel: [w457] -> w167
                  tunnel: w140 -> [w455]
                  tunnel: [w452] -> w165
                  tunnel: "VS filter period (uS)" -> [w418]
                  tunnel: w157 -> [w419]
                  tunnel: w156 -> [w450]
                  tunnel: w155 -> [w443]
                  tunnel: w154 -> [w438]
                  tunnel: w153 -> [w440]
                  shift-right: [w432] -> _
                  shift-left: w152 -> [w445]
                  tunnel: w151 -> [w417]
                  tunnel: w142 -> [w406]
                  tunnel: [w403] -> w145
                  shift-right: [w458] -> w168
                  shift-left: w143 -> [w463]
                  shift-right: [w404] -> w146
                  shift-left: w141 -> [w405]
                  shift-right: [w453] -> w164
                  shift-left: w139 -> [w454]
                  stop <- w465 stop-if-true
                  w430 = T1."Idle"
                  # "Ephys Trigger"
                  # "Pool 100 cycles"
                  # "ADD TRIAL #, Start and end of trial"
                  n232 = node-c288() -> (→"Actual cycle period (uS)":i64)  [unwired: 1 in, 1 out]
                  n233 = local read "Lick reward"() -> (w483:bool)
                  n234 = local read "Reward period (uS)"() -> (w444:u32)
                  n235 = call-poly <vilib>:"DAQmx Read.vi"("task/channels in"=w464, "timeout"=0.1, "error in"=w463) -> ("task out"=w457:refnum<k21>, "data"=w460:dbl[], "error out"=w458:errorcluster)  [unwired: 10 in]
                  n236 = call "Tick Count"() -> ("Tick Count(uSec)"=w491:u32)
                  n237 = Index Array(array=w460, index #1=0 ("index"), index #2=1 ("index"), index #3=2 ("index"), index #4=3 ("index"), index #5=4 ("index")) -> (element #1=w451:dbl, element #2=w459:dbl, element #3=w420:dbl, element #4=w416:dbl, element #5=w423:dbl)
                  n238 = feedback #1(FALSE) -> (w486:bool)
                  n239 = feedback-in #1(w483) -> ()
                  n240 = feedback #2(w491) -> (w492:u32)
                  n241 = feedback-in #2(w491) -> ()
                  n242 = local read "Trial timeout (uS)"() -> (w439:u32)
                  n243 = Greater?(x=w483, y=w486) -> (0:w484:bool)
                  n244 = local read "Pulse delay"() -> (w397:sgl)
                  n245 = Subtract(x=w491, y=w492) -> (x-y=w490:u32)
                  n246 = call "vs digital filter3.vi"("filter period(uSec)"=w418, "vs threshold"=w419, "input"=w420) -> ("output"=w413:bool)  [unwired: 3 in]
                  n247 = To Unsigned Quad Integer(1:w490) -> (0:w489:u64)
                  n248 = Greater?(x=w459, y=w450) -> (0:w412:bool)
                  n249 = feedback #3(u64 0) -> (w488:u64)
                  n250 = Add(x=w489, y=w488) -> (x+y=w442:u64)
                  n251 = Divide(x=w442, y=u64 1000) -> (x/y=w481:dbl)
                  n252 = feedback-in #3(w442) -> ()
                  n253 = call "vs digital filter.vi"("filter period(uSec)"=w418, "vs threshold"=w419, "input"=w451) -> ("output"=w415:bool)  [unwired: 3 in]
                  n254 = feedback #4(w430) -> (w493:T1)
                  n255 = Select(t=T1."Lick reward", s=w484, f=w493) -> (s? t:f=w426:T1)
                  n256 = feedback #5(w430) -> (w431:T1)
                  n257 = Multiply(x=w397, y=sgl 1000.0) -> (x*y=w396:sgl)
                  n258 = local read "ABORT"() -> (w465:bool)
                  n259 = local read "Pulse period (ms)"() -> (w400:sgl)
                  n260 = Build Array(w481, w447, w426, w416) -> (w409:dbl[])
                  n261 = To Single Precision Float(number=w409) -> (single precision float=w410:sgl[])
                  n262 = Multiply(x=w400, y=sgl 1000.0) -> (x*y=w399:sgl)
                  n263 = case shown="\"VS\"" w426 {
                    selector: w426 -> [w508 w517 w532 w557 w567 w590 _ w612 w642 w669 _ w693 w701 w728]
                    tunnel: w448 -> [w509 w525 w540 w561 w584 w595 w606 w625 w646 w671 w686 w695 w713 w731]
                    tunnel: w447 -> [w505 w524 w539 w560 w582 w594 w605 w623 w645 w670 w685 w694 w712 w733]
                    tunnel: w412 -> [_ _ _ _ w570 _ _ _ _ _ _ _ _ w727]
                    tunnel: w446 -> [w504 w523 w538 w559 w574 w593 w602 w622 w632 w667 w683 w692 w707 w726]
                    tunnel: w445 -> [w503 w522 w536 w554 w580 w592 w601 w621 w638 w666 w682 w691 w710 w725]
                    tunnel: w444 -> [_ _ _ _ w578 _ _ _ _ _ _ _ _ _]
                    tunnel: w443 -> [_ _ _ _ _ _ _ w620 _ _ _ _ _ w724]
                    tunnel: w442 -> [_ _ _ w551 w573 _ _ w615 w635 w660 _ _ w704 w720]
                    tunnel: w441 -> [w502 w521 w537 w558 w579 w591 w600 w617 w637 w665 w673 w690 w709 w721]
                    tunnel: w396 -> [_ _ _ w552 _ _ _ _ _ _ _ _ _ _]
                    tunnel: w440 -> [_ _ _ _ _ _ _ _ _ _ _ _ _ _]
                    tunnel: w439 -> [_ _ _ _ _ _ _ _ w641 _ _ _ w705 _]
                    tunnel: w399 -> [_ _ _ _ _ _ _ _ _ w662 _ _ _ _]
                    tunnel: w438 -> [_ _ _ _ _ _ _ _ _ _ _ _ _ _]
                    tunnel: [w509 w525 w540 w561 w584 w595 w606 w624 w646 w671 w686 w695 w713 w732] -> w437
                    tunnel: [w505 w524 w539 w560 w582 w594 w604 w623 w645 w670 w685 w694 w712 w733] -> w436
                    tunnel: [w506 w520 w534 w544 w583 w590 T1."Idle" w614 w644 w653 w684 w693 w703 w729] -> w427
                    tunnel: [FALSE w514 w527 w541 w562 w587 w596 TRUE FALSE FALSE w672 w687 w696 w727] -> w435
                    tunnel: [w504 w523 w538 w559 w572 w593 w602 w622 w632 w667 w683 w692 w700 w726] -> w434
                    tunnel: [w502 w521 w537 w558 w579 w591 w600 w616 w636 w657 w673 w690 w709 w718] -> w433
                    tunnel: [w503 w522 w536 w549 w580 w592 w601 w621 w638 w666 w682 w691 w710 w725] -> w432
                    tunnel: w431 -> [_ _ _ w556 w577 _ _ w627 w643 w668 _ _ w711 w730]
                    tunnel: w415 -> [_ w519 w533 w546 _ _ _ _ _ w656 w681 _ _ _]
                    tunnel: w406 -> [w499 w515 w528 w542 w563 w588 w597 w608 w629 w651 w679 w688 w698 w716]
                    tunnel: w405 -> [w500 w516 w529 w543 w564 w589 w598 w609 w630 w652 w678 w689 w697 w715]
                    tunnel: [w497 w515 w528 w542 w563 w588 w597 w608 w629 w650 w676 w688 w698 w716] -> w403
                    tunnel: [w496 w516 w529 w543 w564 w589 w598 w609 w630 w649 w675 w689 w697 w715] -> w404
                    tunnel: [FALSE w514 w527 w541 w562 w587 w596 FALSE FALSE TRUE w672 w687 w696 FALSE] -> w402
                    frame "Idle", Default {
                      n264 = local read "Start one trial"() -> (w507:bool)
                      n265 = call-poly <vilib>:"DAQmx Write.vi"("task/channels in"=w499, "data"=0.0, "error in"=w500) -> ("task out"=w497:refnum<k21>, "error out"=w496:errorcluster)  [unwired: 10 in, 1 out]
                      n266 = case shown="True" w507 {
                        tunnel: w508 -> [w510 _]
                        tunnel: [w510 w511] -> w506
                        frame False {
                        }
                        frame True {
                          n267 = stacked-sequence {
                            tunnel: [T1."Before VS" _] -> w511
                            frame #0 {
                            }
                            frame #1 {
                              w513 = FALSE
                              n268 = local write "Start one trial"(w513) -> ()
                              n269 = local write "Trial Done"(w513) -> ()
                            }
                          }
                        }
                      }
                    }
                    frame "Before VS" {
                      w514 = FALSE
                      n270 = Select(t=T1."VS", s=w519, f=w517) -> (s? t:f=w520:T1)
                    }
                    frame "VS" {
                      w527 = FALSE
                      n271 = local read "LED?"() -> (w526:bool)
                      n272 = Select(t=T1."VS2", s=w526, f=w532) -> (s? t:f=w531:T1)
                      n273 = Select(t=w531, s=w533, f=T1."Cycle End") -> (s? t:f=w534:T1)
                    }
                    frame "VS2" {
                      w541 = FALSE
                      # "Delay before LED!"
                      # "Punish=LED!!"
                      n274 = Equal?(x=w557, y=w556) -> (x = y?=w555:bool)
                      n275 = Add(x=w551, y=w552) -> (x+y=w553:sgl)
                      n276 = Select(t=w554, s=w555, f=w553) -> (s? t:f=w549:sgl)
                      n277 = Greater?(x=w549, y=w551) -> (0:w550:bool)
                      n278 = Select(t=w557, s=w550, f=T1."Punish") -> (s? t:f=w545:T1)
                      n279 = Select(t=w545, s=w546, f=T1."After VS") -> (s? t:f=w544:T1)
                    }
                    frame "After VS" {
                      w562 = FALSE
                      n280 = Equal?(x=w567, y=w577) -> (x = y?=w575:bool)
                      n281 = Add(x=w578, y=w573) -> (x+y=w576:u64)
                      n282 = Select(t=w574, s=w575, f=w576) -> (s? t:f=w572:u64)
                      n283 = Greater?(x=w572, y=w573) -> (0:w571:bool)
                      n284 = Select(t=T1."Reward", s=w570, f=w567) -> (s? t:f=w568:T1)
                      n285 = Select(t=w568, s=w571, f=T1."Cycle End") -> (s? t:f=w581:T1)
                      n286 = case shown="True" "Automatic reward" {
                        tunnel: [w585 T1."Reward"] -> w583
                        tunnel: w581 -> [w585 _]
                        frame False {
                        }
                        frame True {
                        }
                      }
                    }
                    frame "Wait for lever press" {
                      w587 = FALSE
                    }
                    frame "Cycle End" {
                      w596 = FALSE
                      n287 = Increment(x=w605) -> (x+1=w604:i32)
                      n288 = local write "Trial Done"(TRUE) -> ()
                    }
                    frame "Reward" {
                      n289 = Add(x=w620, y=w615) -> (x+y=w619:u64)
                      n290 = Increment(x=w625) -> (x+1=w626:i32)
                      n291 = Equal?(x=w612, y=w627) -> (x = y?=w618:bool)
                      n292 = Select(t=w617, s=w618, f=w619) -> (s? t:f=w616:sgl)
                      n293 = Select(t=w625, s=w618, f=w626) -> (s? t:f=w624:i32)
                      "# of rewards" <- w624
                      n294 = Greater?(x=w616, y=w615) -> (0:w613:bool)
                      n295 = Select(t=w612, s=w613, f=T1."Cycle End") -> (s? t:f=w614:T1)
                    }
                    frame "Reward Refractory" {
                      n296 = Equal?(x=w642, y=w643) -> (x = y?=w639:bool)
                      n297 = Add(x=w635, y=w641) -> (x+y=w640:u64)
                      n298 = Select(t=w637, s=w639, f=w640) -> (s? t:f=w636:sgl)
                      n299 = Greater?(x=w636, y=w635) -> (0:w634:bool)
                      n300 = Select(t=w642, s=w634, f=T1."Cycle End") -> (s? t:f=w644:T1)
                    }
                    frame "Punish" {
                      # "=LED!!"
                      n301 = Equal?(x=w669, y=w668) -> (x = y?=w664:bool)
                      n302 = local read "Pulse amp 0"() -> (w648:sgl)
                      n303 = Add(x=w660, y=w662) -> (x+y=w663:sgl)
                      n304 = Select(t=w665, s=w664, f=w663) -> (s? t:f=w657:sgl)
                      n305 = call-poly <vilib>:"DAQmx Write.vi"("task/channels in"=w651, "data"=w648, "error in"=w652) -> ("task out"=w650:refnum<k21>, "error out"=w649:errorcluster)  [unwired: 10 in, 1 out]
                      n306 = Greater?(x=w657, y=w660) -> (0:w661:bool)
                      n307 = Select(t=w669, s=w661, f=T1."Punish Refractory") -> (s? t:f=w654:T1)
                      n308 = Select(t=w654, s=w656, f=T1."Punish Refractory") -> (s? t:f=w653:T1)
                    }
                    frame "Punish Refractory" {
                      w672 = FALSE
                      # "Possibly code LED refractory period"
                      # "STOP LED HERE!"
                      n309 = call-poly <vilib>:"DAQmx Write.vi"("task/channels in"=w679, "data"=0.0, "error in"=w678) -> ("task out"=w676:refnum<k21>, "error out"=w675:errorcluster)  [unwired: 10 in, 1 out]
                      n310 = Select(t=T1."VS", s=w681, f=T1."After VS") -> (s? t:f=w684:T1)
                    }
                    frame "Exit" {
                      w687 = FALSE
                    }
                    frame "Timeout" {
                      w696 = FALSE
                      # "Can be used for pre-VS state for suppressing LED"
                      n311 = Equal?(x=w701, y=w711) -> (x = y?=w708:bool)
                      n312 = Add(x=w704, y=w705) -> (x+y=w706:u64)
                      n313 = Select(t=w707, s=w708, f=w706) -> (s? t:f=w700:u64)
                      n314 = Greater?(x=w700, y=w704) -> (0:w702:bool)
                      n315 = Select(t=w701, s=w702, f=T1."Cycle End") -> (s? t:f=w703:T1)
                    }
                    frame "Lick reward" {
                      n316 = Equal?(x=w728, y=w730) -> (x = y?=w723:bool)
                      n317 = Add(x=w724, y=w720) -> (x+y=w722:u64)
                      n318 = Select(t=w721, s=w723, f=w722) -> (s? t:f=w718:sgl)
                      n319 = Greater?(x=w718, y=w720) -> (0:w719:bool)
                      n320 = case shown="True" w727 {
                        tunnel: [w734 w736] -> w732
                        tunnel: w731 -> [w734 w735]
                        frame False {
                        }
                        frame True {
                          n321 = Increment(x=w735) -> (x+1=w736:i32)
                        }
                      }
                      n322 = Select(t=w728, s=w719, f=T1."Reward Refractory") -> (s? t:f=w729:T1)
                    }
                  }
                  n323 = local read "Manually give water"() -> (w482:bool)
                  n324 = shared-variable "My Computer\\Network variables.lvlib\\stop - network"() -> (w494:bool)  [unwired: 1 in, 1 out]
                  n325 = Select(t=T1."Exit", s=w494, f=w427) -> (s? t:f=w449:T1)
                  n326 = feedback-in #4(w449) -> ()
                  n327 = feedback-in #5(w449) -> ()
                  n328 = Or(x=w482, y=w435) -> (x .or. y?=w411:bool)
                  n329 = Build Array(w413, w402, w411) -> (w468:bool[])
                  n330 = Boolean Array To Number(Boolean array=w468) -> (number=w407:u32)
                  n331 = To Single Precision Float(number=w407) -> (single precision float=w408:sgl)
                  n332 = Build Array (concatenate)(w410, w408) -> (w467:sgl[])
                  n333 = Build Array (concatenate)(w479, w467) -> (w475:sgl[])
                  n334 = Array Size(array=w475) -> (size(s)=w470:i32)
                  n335 = Equal?(x=w470, y=w417) -> (x = y?=w469:bool)
                  n336 = case shown="True" w469 {
                    tunnel: w478 -> [_ w749]
                    tunnel: [w739 w748] -> w477
                    tunnel: w476 -> [w739 w746]
                    tunnel: w475 -> [w738 w743]
                    tunnel: [w738 sgl[] [] ("array type (2D Dbl)")] -> w474
                    tunnel: w473 -> [_ w742]
                    tunnel: w472 -> [w737 w741]
                    tunnel: [w737 w740] -> w471
                    frame False {
                    }
                    frame True {
                      n337 = RT FIFO Write(0:w749, 1:w743, 2:10 ("timeout in ms (0)"), 3:w746) -> (11:w748:errorcluster)  [unwired: 1 in, 3 out]
                      n338 = RT FIFO Write(0:w742, 1:w743, 2:10 ("timeout in ms (0)"), 3:w741) -> (11:w740:errorcluster)  [unwired: 1 in, 3 out]
                    }
                  }
                  n339 = call "vs digital filter2.vi"("filter period(uSec)"=w418, "vs threshold"=w419, "input"=w423) -> ("output"=w414:bool)  [unwired: 3 in]
                  n340 = Build Array(w411, w414, w413) -> (w456:bool[])
                  n341 = node-c288() -> ()  [unwired: 3 in, 1 out]
                  n342 = call-poly <vilib>:"DAQmx Write.vi"("task/channels in"=w455, "data"=w456, "error in"=w454) -> ("task out"=w452:refnum<k21>, "error out"=w453:errorcluster)  [unwired: 10 in, 1 out]
                }
                n343 = node-c288(w210) -> (w203:errorcluster)
                n344 = call <vilib>:"DAQmx Stop Task.vi"("task/channels in"=w145, "error in"=w146) -> ("error out"=w147:errorcluster)  [unwired: 12 in, 1 out]
                n345 = call <vilib>:"DAQmx Stop Task.vi"("task/channels in"=w167, "error in"=w168) -> ("error out"=w166:errorcluster)  [unwired: 12 in, 1 out]
                n346 = Merge Errors(w197, w200, w192, w191) -> (w199:errorcluster)
                n347 = Build Array(w159, w159, w159) -> (w161:bool[])
                n348 = call-poly <vilib>:"DAQmx Write.vi"("task/channels in"=w165, "data"=w161, "error in"=w164) -> ("task out"=w163:refnum<k21>, "error out"=w162:errorcluster)  [unwired: 10 in, 1 out]
                n349 = call <vilib>:"DAQmx Stop Task.vi"("task/channels in"=w163, "error in"=w162) -> ("error out"=w181:errorcluster)  [unwired: 12 in, 1 out]
                n350 = Merge Errors(w166, w181, w147) -> (w201:errorcluster)
                n351 = stacked-sequence {
                  tunnel: w218 -> [w765]
                  tunnel: w219 -> [w764]
                  tunnel: w205 -> [w762]
                  tunnel: w204 -> [w761]
                  tunnel: w203 -> [w760]
                  tunnel: w201 -> [w759]
                  tunnel: w199 -> [w758]
                  frame #0 {
                    n352 = Merge Errors(w760, w761, w765, w764, w762, w759, w758) -> (w763:errorcluster)
                    "error out" <- w763
                    n353 = call <vilib>:"Simple Error Handler.vi"("error in (no error)"=w763) -> ()  [unwired: 4 in, 5 out]
                  }
                }
              }
            }
          }
          frame #2 {
            n354 = Wait (ms)(milliseconds to wait=u32 50) -> ()  [unwired: 1 out]
          }
        }
      }
      n355 = UDP Close(connection ID=w2, 8:w3) -> (error out=w1:errorcluster)  [unwired: 1 out]
      n356 = call <vilib>:"Simple Error Handler.vi"("error in (no error)"=w1) -> ()  [unwired: 4 in, 5 out]
    }
    frame #1 {
      w1000 = FALSE
      n357 = local write "Busy"(w1000) -> ()
      n358 = local write "ABORT"(w1000) -> ()
      n359 = local write "Initial data received"(w1000) -> ()
      n360 = local write "Stop state"(w1000) -> ()
    }
  }
